vi "Robot_Enabled.vi"() -> (3 "Robot Enabled":bool)   [LabVIEW 2023]
doc: "Return TRUE if robot is enabled."
uses:
  <vilib>/Rock Robotics/WPI/DriverStation/WPI_DriverStationRobotMode2.ctl
  LED_TEST/Robot Global Data.vi
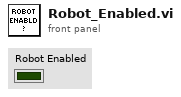
[diagram p1: front panel]
types:
  T1 = typedef "WPI_DriverStationRobotMode2.ctl" = enum16{"Autonomous Disabled", "Autonomous Enabled", "Teleop Disabled", "Teleop Enabled", "Disconnected", "Finish", "Test Disabled", "Test Enabled", "Emergency Stopped"}
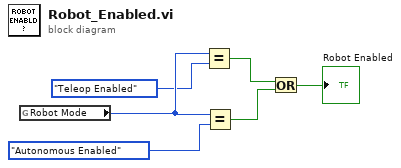
[diagram p0: block diagram]
diagram:
  n1 = global read "Robot Global Data.vi" "Robot Mode"() -> (w4:T1)
  n2 = Equal?(x=w4, y=WPI_DriverStationRobotMode2."Teleop Enabled") -> (x = y?=w5:bool)
  n3 = Equal?(x=w4, y=WPI_DriverStationRobotMode2."Autonomous Enabled") -> (x = y?=w6:bool)
  n4 = Or(x=w5, y=w6) -> (x .or. y?=→"Robot Enabled":bool)
